vi "Test Results Stacked Bar Graph Example.vi"() -> ()   [LabVIEW 2019]
uses:
  Python Visualizations Library/pieplot_labels.ctl
  Python Visualizations Library/Python Visualizations.lvlib
panel:
  out "Test Results Stacked Bar Graph":picture
  in  "Test Results":T1={"# of passing results"=[30.0, 35.0, 40.0, 50.0, 58.0], "# of failing results"=[10.0, 9.0, 7.0, 5.0, 2.0], "# of error results"=[5.0, 5.0, 5.0, 2.0, 1.0]}
  in  "Labels":T2={"dataset labels"=["Jan", "Feb", "Mar", "April", "May"], "title"="Test Results 2019"}
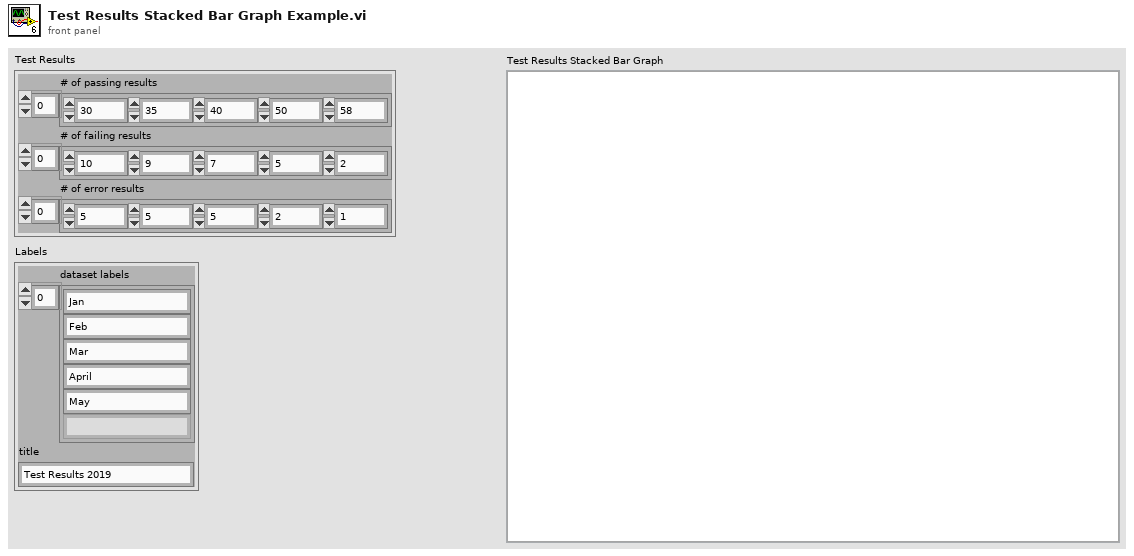
[diagram p1: front panel]
types:
  T1 = cluster{"# of passing results":dbl[], "# of failing results":dbl[], "# of error results":dbl[]}
  T2 = typedef "Python Visualizations.lvlib/pieplot_labels.ctl" = cluster{"dataset labels":string[], "title":string}
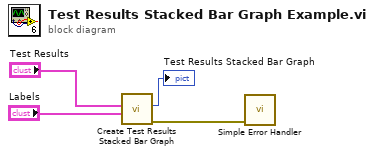
[diagram p0: block diagram]
diagram:
  n1 = call "Create Test Results Stacked Bar Graph.vi"("labels"="Labels", "test results"="Test Results") -> ("error out"=w1:errorcluster, "test results stacked bar graph"=→"Test Results Stacked Bar Graph":picture)  [unwired: 8 in]
  n2 = call <vilib>:"Simple Error Handler.vi"("error in (no error)"=w1) -> ()  [unwired: 4 in, 5 out]
